vi "ClassAttributes_GetClassAttributes_6x8x6.vi"(0 "reference in":refnum<class>, 1 "OnlyGetDvrReference(False)":bool, 5 "error in":errorcluster) -> (14 "reference out":refnum<class>, 15 "Class attribute":T1, 17 "Class attribute Reference":refnum<data-value>, 19 "error out":errorcluster)   [LabVIEW 2020]
doc: "Returns the class attributes of this class or a sub class. If reference is wired, the class attributes of the class (or sub class) will be returned else the class attributes will default to this class.\n\nIf the data is currently locked for modification, 'Attributes locked?' will return TRUE. If reference is wired, the class attributes of this class (or sub class) will be returned else the class attributes of this class."
uses:
  <resource>/Framework/Providers/Open_GDS/ClassProviders/DesignPatterns/ClassAttributes/ClassAttributes_SubVIs/ClassAttributes_ClassAttributes.ctl
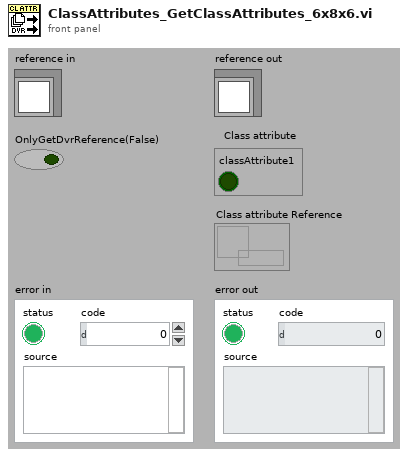
[diagram p1: front panel]
types:
  T1 = typedef "ClassAttributes_ClassAttributes.ctl" = cluster{"classAttribute1":bool}
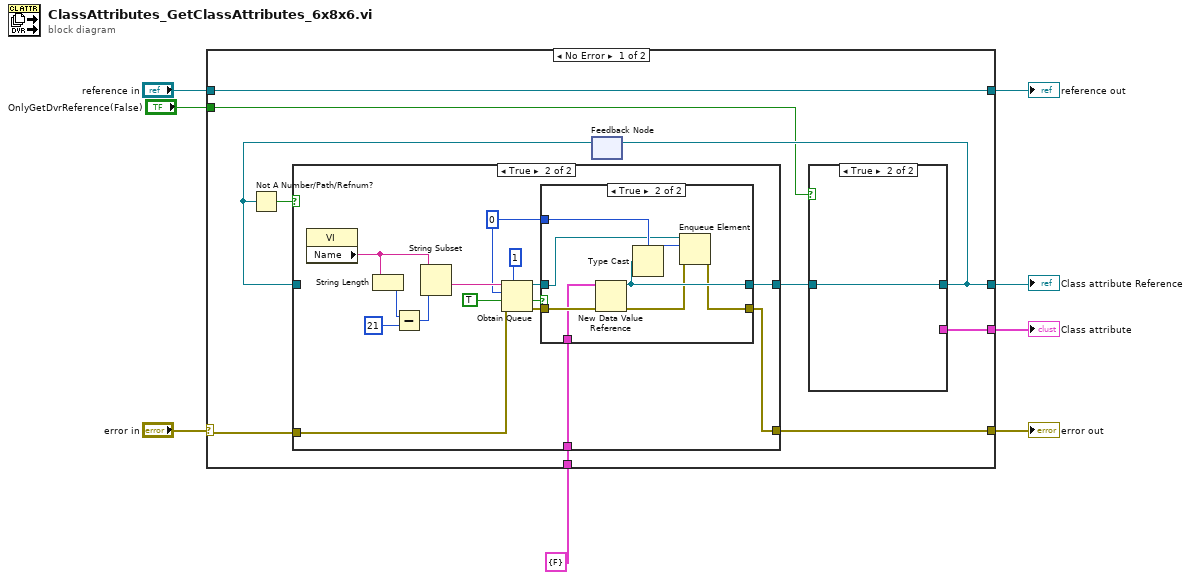
[diagram p0: block diagram]
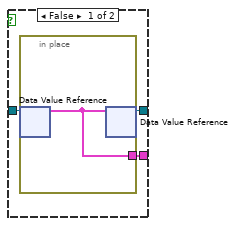
[diagram p2: hidden frame]
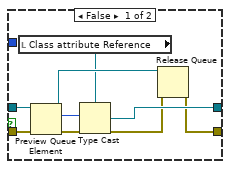
[diagram p4: hidden frame]
diagram:
  n1 = case shown="No Error" "error in" {
    selector: "error in" -> [w16 w57]
    tunnel: [w18 w58] -> w8
    tunnel: [w15 w57] -> w7
    tunnel: "reference in" -> [w18 w58]
    tunnel: T1 {"classAttribute1"=FALSE} ("Class attributes") -> [w17 _]
    tunnel: [w13 _] -> w3
    tunnel: [w14 _] -> w2
    tunnel: "OnlyGetDvrReference(False)" -> [w9 _]
    frame No Error {
      n2 = feedback #1() -> (w10:refnum<data-value>)  [unwired: 1 in]
      n3 = Not A Number/Path/Refnum?(number/path/refnum=w10) -> (NaN/Path/Refnum?=w11:bool)
      n4 = case shown="True" w11 {
        tunnel: w17 -> [_ w40]
        tunnel: w16 -> [w24 w39]
        tunnel: [w24 w38] -> w15
        tunnel: [w25 w28] -> w12
        tunnel: w10 -> [w25 _]
        frame False {
        }
        frame True {
          w27 = u32 0 ("max queue size (-1, unlimited)")
          n5 = property class="VI"() -> ("Name"=w26:string)  [unwired: 2 in, 2 out]
          n6 = String Length(string=w26) -> (length=w37:i32)
          n7 = Subtract(x=w37, y=21) -> (x-y=w35:i32)
          n8 = String Subset(string=w26, length (rest)=w35) -> (substring=w34:string)  [unwired: 1 in]
          n9 = Obtain Queue(max queue size (-1, unlimited)=1, name (unnamed)=w34, element data type=w27, create if not found? (T)=TRUE, error in (no error)=w39) -> (queue out=w29:refnum<queue>, created new?=w31:bool, error out=w30:errorcluster)
          n10 = case shown="True" w31 {
            tunnel: w30 -> [w48 w56]
            tunnel: w40 -> [_ w55]
            tunnel: w29 -> [w47 w52]
            tunnel: [w45 w54] -> w28
            tunnel: [w42 w49] -> w38
            tunnel: w27 -> [_ w53]
            frame False {
              n11 = local read "Class attribute Reference"() -> (w41:refnum<data-value>)
              n12 = Preview Queue Element(queue=w47, error in (no error)=w48) -> (queue out=w44:refnum<queue>, element=w46:u32, error out=w43:errorcluster)  [unwired: 1 in, 1 out]
              n13 = Type Cast(type=w41, x=w46) -> (*(type *) &x=w45:refnum<data-value>)
              n14 = Release Queue(queue=w44, error in (no error)=w43) -> (error out=w42:errorcluster)  [unwired: 1 in, 2 out]
            }
            frame True {
              n15 = New Data Value Reference(data value=w55, error in=w56) -> (data value reference=w54:refnum<data-value>, error out=w50:errorcluster)
              n16 = Type Cast(type=w53, x=w54) -> (*(type *) &x=w51:u32)
              n17 = Enqueue Element(queue=w52, element=w51, error in (no error)=w50) -> (error out=w49:errorcluster)  [unwired: 1 in, 2 out]
            }
          }
        }
      }
      n18 = case shown="True" w9 {
        tunnel: [w21 _] -> w14
        tunnel: [w20 w23] -> w13
        tunnel: w12 -> [w19 w23]
        frame False {
          n19 = in-place {
            in-place-border: [w22] -> w21
            n20 = in-place-dvr #2(w19) -> (w22:T1)  [unwired: 1 out]
            n21 = in-place-dvr #2(w22) -> (w20:refnum<data-value>)  [unwired: 1 out]
          }
        }
        frame True {
        }
      }
      n22 = feedback-in #1(w13) -> ()
    }
    frame Error {
    }
  }
  "error out" <- w7
  "reference out" <- w8
  "Class attribute" <- w2
  "Class attribute Reference" <- w3
